vi "LabVIEW Basics #4 - Ultrasonic Sensor DAQ.vi"() -> ()   [LabVIEW 2019]
uses:
  <vilib>/MakerHub/LINX/Public/Utilities/Open Serial.vi
  <vilib>/MakerHub/LINX/Public/Sensors/Motion/Servo/Servo Open One Channel.vi
  <vilib>/MakerHub/LINX/Public/Sensors/Motion/Servo/Servo Set Pulse Width One Channel.vi
  <vilib>/MakerHub/LINX/Public/Sensors/Motion/Servo/Servo Close One Channel.vi
  <vilib>/MakerHub/LINX/LMH-LINX.lvlib
  <vilib>/MakerHub/LINX/Public/Sensors/Motion/Servo/Servo.lvlib
  <vilib>/MakerHub/LINX/Public/Sensors/Distance/Ultrasonic/Ultrasonic.lvlib
  <vilib>/ptbypt/NI_PtbyPt.lvlib
panel:
  out "Angle (Deg)":dbl(knob) caption="Angle(Deg)" scale=0.0..180.0
  out "Slide":dbl(slide) scale=2.0..400.0
  out "Distance (cm)":dbl format="%#_3g"
  out "Device Name":string
  in  "Stop":bool
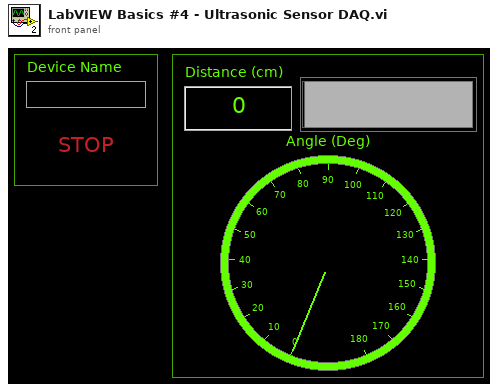
[diagram p1: front panel]
types:
  T1 = typedef "LMH-LINX.lvlib/LINX Ref.ctl" = cluster{"IO":T2, "Interface":T3, "LINX Device Config":T4}
  T2 = typedef "LMH-LINX.lvlib/Platform.ctl" = enum16{"Remote", "Local"}
  T3 = typedef "LMH-LINX.lvlib/Interface.ctl" = enum16{"Serial", "TCP"}
  T4 = typedef "LMH-LINX.lvlib/Device.lvlib/LINX Device Config.ctl" = cluster{"Interface":T3, "COM Port":refnum<visa-resource-name>, "TCP Configuration":T5, "Device Family":u8, "Device ID":u8, "Device Name":string, "TCP Ref":refnum<k5>, "Channels":T6}
  T5 = typedef "LMH-LINX.lvlib/Device.lvlib/TCP Config.ctl" = cluster{"IP Address":string, "Port":u16}
  T6 = typedef "LMH-LINX.lvlib/Channels.ctl" = cluster{"DI":u8[], "DO":u8[], "AI":u8[], "AO":u8[], "PWM":u8[], "QE":u8[], "UART":u8[], "I2C 2":u8[], "SPI":u8[], "CAN":u8[], "Servo":u8[], "AI Ref (V)":dbl, "AI Resolution (Bits)":u8, "AO Ref (V)":dbl, "AO Resolution (Bits)":u8}
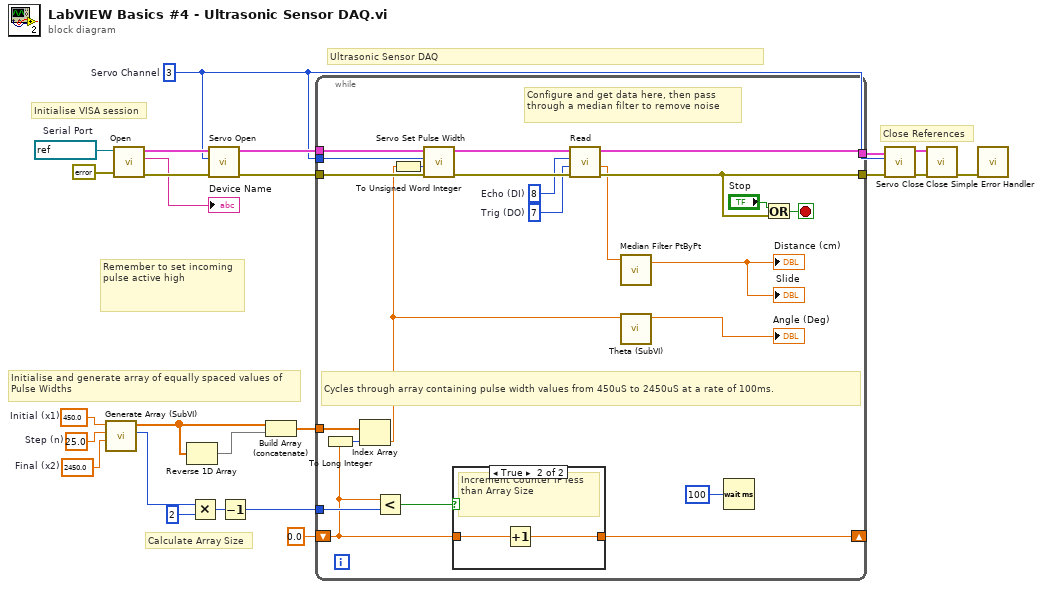
[diagram p0: block diagram]
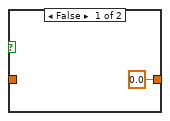
[diagram p2: hidden frame]
diagram:
  w12 = 2450.0  # Final (x2)
  w11 = 25.0  # Step (n)
  w10 = 450.0  # Initial (x1)
  w15 = u8 3  # Servo Channel
  w24 = refnum<visa-resource-name> "COM6"  # Serial Port
  # "Remember to set incoming pulse active high"
  # "Close References"
  # "Calculate Array Size"
  # "Initialise and generate array of equally spaced values of Pulse Widths"
  # "Initialise VISA session"
  # "Ultrasonic Sensor DAQ"
  n1 = call "Generate Array (SubVI).vi"("Final"=w12, "Step"=w11, "Initial"=w10) -> ("Array size"=w5:i32, "Array out"=w8:dbl[])  [unwired: 6 in, 1 out]
  n2 = call-poly <vilib>:"Open.vi"("Error In"=errorcluster {"status"=FALSE, "code"=0, "source"=""}, "Serial Port"=w24) -> ("Error Out"=w20:errorcluster, "Device Name"=→"Device Name":string, "LINX Resource"=w21:T1)  [unwired: 7 in]
  n3 = Reverse 1D Array(array=w8) -> (reversed array=w7:dbl[])
  n4 = Multiply(x=w5, y=2) -> (x*y=w6:i32)
  n5 = call-poly <vilib>:"Servo Open.vi"("Error In"=w20, "Servo Channel"=w15, "LINX Resource"=w21) -> ("Error Out"=w18:errorcluster, "LINX Resource"=w19:T1)  [unwired: 7 in]
  n6 = Decrement(x=w6) -> (x-1=w13:i32)
  n7 = Build Array (concatenate)(w8, w7) -> (w9:dbl[])
  n8 = while {
    tunnel: [w39] -> w23
    tunnel: [w33] -> w22
    tunnel: w19 -> [w41]
    tunnel: w18 -> [w42]
    tunnel: w15 -> [w46]
    tunnel: w9 -> [w45]
    shift-right: [w35] -> _
    shift-left: 0.0 -> [w30]
    tunnel: w13 -> [w44]
    stop <- w47 stop-if-true
    w36 = u8 7  # Trig (DO)
    w37 = u8 8  # Echo (DI)
    # "Configure and get data here, then pass through a median filter to remove noise"
    # "Cycles through array containing pulse width values from 450uS to 2450uS at a rate of 100ms."
    n9 = To Long Integer(number=w30) -> (32bit integer=w29:i32)
    n10 = Index Array "Index Array"(array=w45, index=w29) -> (element=w27:dbl)
    n11 = Less?(x=w30, y=w44) -> (x < y?=w43:bool)
    n12 = To Unsigned Word Integer(number=w27) -> (unsigned 16bit integer=w28:u16)
    n13 = call-poly <vilib>:"Servo Set Pulse Width.vi"("Error In"=w42, "Pulse Width (uS)"=w28, "Servo Channel"=w46, "LINX Resource"=w41) -> ("Error Out"=w38:errorcluster, "LINX Resource"=w40:T1)  [unwired: 6 in]
    n14 = case shown="True" w43 {
      tunnel: [0.0 w50] -> w35
      tunnel: w30 -> [_ w49]
      frame False {
      }
      frame True {
        # "Increment Counter IF less than Array Size"
        n15 = Increment(x=w49) -> (x+1=w50:dbl)
      }
    }
    n16 = call <vilib>:"Read.vi"("Error In"=w38, "DO Channel"=w36, "DI Channel"=w37, "LINX Resource"=w40) -> ("Error Out"=w33:errorcluster, "Centimeters"=w32:dbl, "LINX Resource"=w39:T1)  [unwired: 4 in, 1 out]
    n17 = call <vilib>:"Median Filter PtByPt.vi"("x"=w32) -> ("Filtered x"=→"Distance (cm)" →"Slide":dbl)  [unwired: 3 in, 1 out]
    n18 = call "Theta (SubVI).vi"("PWM"=w27) -> ("Theta"=→"Angle (Deg)":dbl)  [unwired: 9 in, 1 out]
    n19 = Wait (ms)(milliseconds to wait=u32 100 ("Slide")) -> ()  [unwired: 1 out]
    n20 = Or(x="Stop", y=w33) -> (x .or. y?=w47:bool)
  }
  n21 = call-poly <vilib>:"Servo Close.vi"("Error In"=w22, "Servo Channel"=w15, "LINX Resource"=w23) -> ("Error Out"=w17:errorcluster, "LINX Resource"=w16:T1)  [unwired: 7 in]
  n22 = call <vilib>:"Close.vi"("Error In"=w17, "LINX Resource"=w16) -> ("Error Out"=w1:errorcluster)  [unwired: 9 in]
  n23 = call <vilib>:"Simple Error Handler.vi"("error in (no error)"=w1) -> ()  [unwired: 4 in, 5 out]
